vi "FlattenImageToString.vi"(6 "Quality":i32=750, 7 "Flatten with Process-Unique Name (F)":bool, 8 "error in":errorcluster, 9 "Type of Flatten":T1 items=["Image", "Image and Vision Info", "Reference to Image"], 10 "Compression":T2 items=["None", "JPEG", "PACKED BINARY"], 11 "Image Reference In":T3) -> (0 "error out":errorcluster, 2 "DataString":string, 3 "Image Reference Out":T3)   [LabVIEW 2024, in "OpenLvVision_Image.lvlib" / "DataAccess.lvlib"]
doc: "Returns the image data as a binary string."
uses:
  DataAccess.lvlib
  Management/TypeDef/Image.ctl
  TypeDef/FlattenCompression.ctl
  TypeDef/TypeOfFlatten.ctl
  Management/Management.lvlib
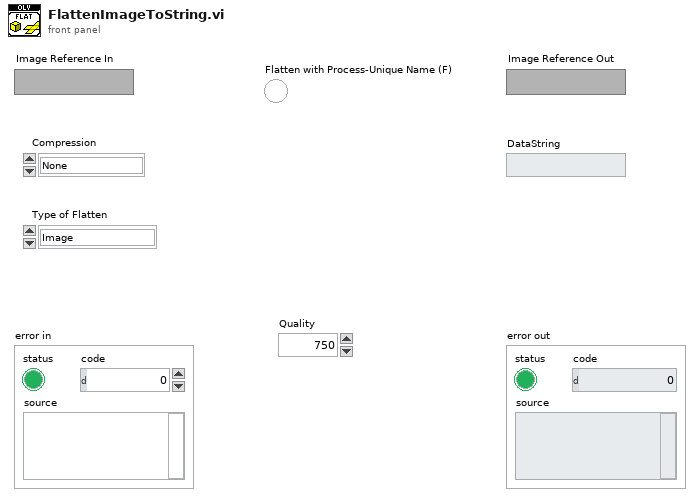
[diagram p1: front panel]
types:
  T1 = typedef "OpenLvVision_Image.lvlib/DataAccess.lvlib/TypeOfFlatten.ctl" = i32
  T2 = typedef "OpenLvVision_Image.lvlib/DataAccess.lvlib/FlattenCompression.ctl" = i32
  T3 = typedef "OpenLvVision_Image.lvlib/Management.lvlib/Image.ctl" = refnum<image>
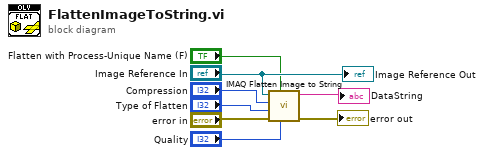
[diagram p0: block diagram]
diagram:
  n1 = call "IMAQ Flatten Image to String"("Quality (750)"="Quality", "Flatten with Process-Unique Name (F)"="Flatten with Process-Unique Name (F)", "error in (no error)"="error in", "Type of Flatten (Image and Vision Info)"="Type of Flatten", "Compression (None)"="Compression", "Image"="Image Reference In") -> ("error out"=→"error out":errorcluster, "Data String"=→"DataString":string)  [unwired: 4 in]
  "Image Reference Out" <- "Image Reference In"
